vi "KeyenceCVX.Main.Init.vi"(8 "error in":errorcluster, 10 "restart":bool=TRUE, 11 "Data":T1) -> (0 "error out":errorcluster, 3 "Data out":T1)   [LabVIEW 2016]
uses:
  KeyenceCVX.Data.ctl
  KeyenceCVX.Data.Status.ctl
  KeyenceCVX.Data.Status.State.ctl
  KeyenceCVX.Data.Sets.ctl
  KeyenceCVX.CodeDetails.ctl
  private/controls/RunMode.ctl
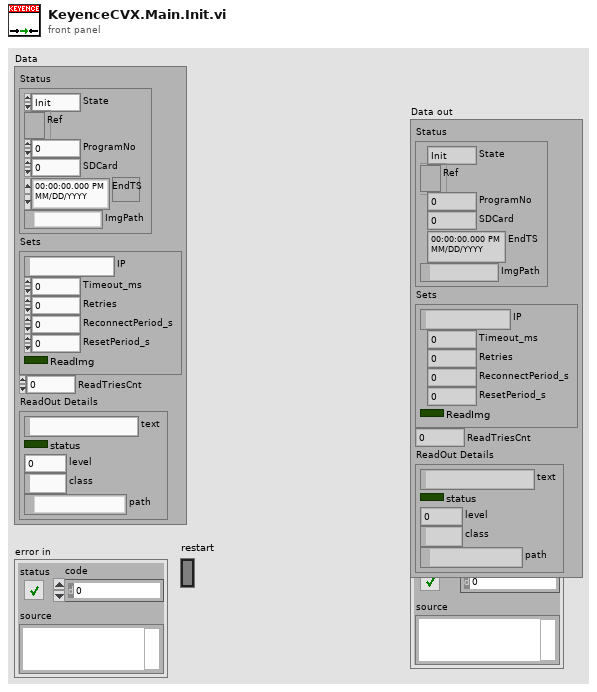
[diagram p1: front panel]
types:
  T1 = typedef "KeyenceCVX.Data.ctl" = cluster{"Status":T2, "Sets":T4, "ReadTriesCnt":u8, "ReadOut Details":T5}
  T2 = typedef "KeyenceCVX.Data.Status.ctl" = cluster{"State":T3, "Ref":refnum<k5>, "ProgramNo":u16, "SDCard":u8, "EndTS":timestamp, "ImgPath":path}
  T3 = typedef "KeyenceCVX.Data.Status.State.ctl" = enum16{"Init", "Reset", "Idle", "Scan"}
  T4 = typedef "KeyenceCVX.Data.Sets.ctl" = cluster{"IP":string, "Timeout_ms":i32, "Retries":i32, "ReconnectPeriod_s":i32, "ResetPeriod_s":i32, "ReadImg":bool}
  T5 = typedef "KeyenceCVX.CodeDetails.ctl" = cluster{"text":string, "status":bool, "level":u8, "class":string, "path":path}
  T6 = typedef "RunMode.ctl" = enum16{"SETUP", "RUN"}
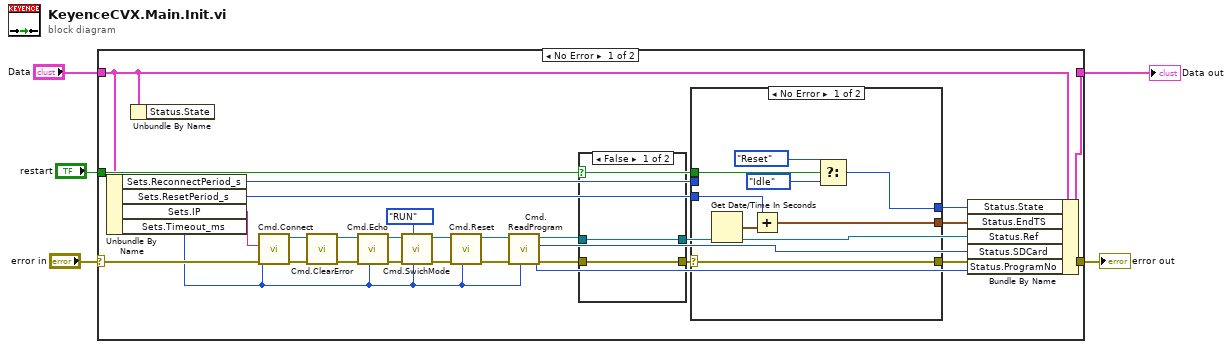
[diagram p0: block diagram]
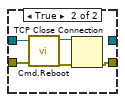
[diagram p2: hidden frame]
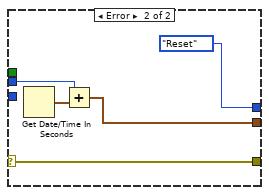
[diagram p3: hidden frame]
diagram:
  n1 = case shown="No Error" "error in" {
    selector: "error in" -> [w24 w55]
    tunnel: [w26 w55] -> w4
    tunnel: "Data" -> [w23 w54]
    tunnel: [w33 w54] -> w1
    tunnel: "restart" -> [w27 _]
    frame No Error {
      n2 = Unbundle By Name(w23) -> ("Sets.ReconnectPeriod_s"=w29:i32, "Sets.ResetPeriod_s"=w30:i32, "Sets.IP"=w25:string, "Sets.Timeout_ms"=w10:i32)
      n3 = Unbundle By Name(w23) -> ()  [unwired: 1 out]
      n4 = call "Cmd.Connect.vi"("error in (no error)"=w24, "Timeout [ms] (1000)"=w10, "IP"=w25) -> ("error out"=w7:errorcluster, "connection ID out"=w9:refnum<k5>)  [unwired: 7 in]
      n5 = call "Cmd.ClearError.vi"("error in"=w7, "cID in"=w9) -> ("error out"=w6:errorcluster, "cID out"=w8:refnum<k5>)  [unwired: 8 in]
      n6 = call "Cmd.Echo.vi"("Timeout [ms] (1000)"=w10, "error in"=w6, "cID in"=w8) -> ("error out"=w15:errorcluster, "cID out"=w16:refnum<k5>)  [unwired: 7 in]
      n7 = call "Cmd.SwichMode.vi"("Timeout [ms] (1000)"=w10, "RunMode"=RunMode."RUN", "error in"=w15, "cID in"=w16) -> ("error out"=w13:errorcluster, "cID out"=w14:refnum<k5>)  [unwired: 6 in]
      n8 = call "Cmd.Reset.vi"("Timeout [ms] (1000)"=w10, "error in"=w13, "cID in"=w14) -> ("error out"=w11:errorcluster, "cID out"=w12:refnum<k5>)  [unwired: 7 in]
      n9 = call "Cmd.ReadProgram.vi"("Timeout [ms] (1000)"=w10, "error in"=w11, "cID in"=w12) -> ("error out"=w19:errorcluster, "ProgramNumber"=w20:u16, "SDCard"=w21:u8, "cID out"=w18:refnum<k5>)  [unwired: 5 in]
      n10 = case shown="False" w27 {
        tunnel: w19 -> [w35 w39]
        tunnel: [w35 w40] -> w31
        tunnel: w18 -> [w34 w38]
        tunnel: [w34 _] -> w22
        frame False {
        }
        frame True {
          n11 = call "Cmd.Reboot.vi"("error in"=w39, "cID in"=w38) -> ("error out"=w36:errorcluster, "cID out"=w37:refnum<k5>)  [unwired: 8 in]
          n12 = TCP Close Connection(connection ID=w37, error in (no error)=w36) -> (error out=w40:errorcluster)  [unwired: 1 in, 1 out]
        }
      }
      n13 = case shown="No Error" w31 {
        selector: w31 -> [w43 w49]
        tunnel: [w45 KeyenceCVX.Data.Status.State."Reset" ("State")] -> w32
        tunnel: w30 -> [w47 _]
        tunnel: w29 -> [_ w52]
        tunnel: [w46 w50] -> w28
        tunnel: w27 -> [w44 _]
        tunnel: [w43 w49] -> w26
        frame No Error {
          n14 = Get Date/Time In Seconds() -> (seconds since 1Jan1904=w48:timestamp)
          n15 = Add(x=w47, y=w48) -> (x+y=w46:timestamp)
          n16 = Select(t=KeyenceCVX.Data.Status.State."Reset" ("State"), s=w44, f=KeyenceCVX.Data.Status.State."Idle" ("State")) -> (s? t:f=w45:T3)
        }
        frame Error {
          n17 = Get Date/Time In Seconds() -> (seconds since 1Jan1904=w51:timestamp)
          n18 = Add(x=w52, y=w51) -> (x+y=w50:timestamp)
        }
      }
      n19 = Bundle By Name(cluster=w23, "Status.State"=w32, "Status.EndTS"=w28, "Status.Ref"=w22, "Status.SDCard"=w21, "Status.ProgramNo"=w20) -> (w33:T1)
    }
    frame Error {
    }
  }
  "error out" <- w4
  "Data out" <- w1
